vi "EventCounting_GetValue.vi"(3 "error in (no error)":errorcluster, 5 "Task ID":u32) -> (0 "error out":errorcluster, 1 "event count":u32, 2 "Task ID":u32)   [LabVIEW 2015]
uses:
  Windows/System32/AdvLvDaq.dll
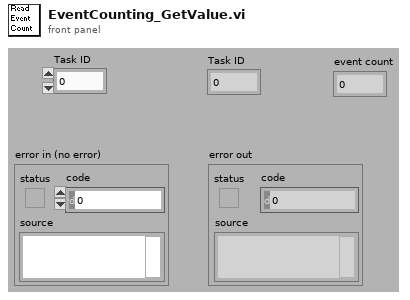
[diagram p1: front panel]
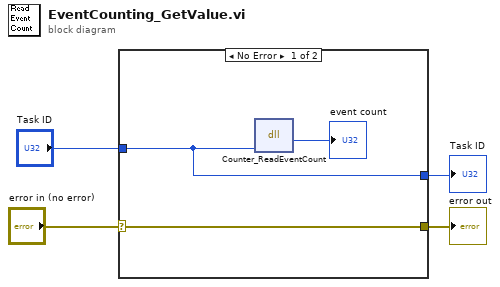
[diagram p0: block diagram]
diagram:
  n1 = case shown="No Error" "error in (no error)" {
    selector: "error in (no error)" -> [w6 w8]
    tunnel: [w6 w8] -> w3
    tunnel: "Task ID" -> [w5 w9]
    tunnel: [w5 w9] -> w1
    frame No Error {
      n2 = dll-call lib="C:/Windows/System32/AdvLvDaq.dll" fn="Counter_ReadEventCount"("taskId"=w5) -> ("return type"=→"event count":u32)  [unwired: 4 in, 2 out]
    }
    frame Error {
    }
  }
  "error out" <- w3
  "Task ID" <- w1
